vi "Open From Disk.vi"(8 "error in (no error)":errorcluster, 9 "Mode":T1, 10 "Path":path, 11 "Database Manager in":refnum<class "Database Manager.lvclass">) -> (0 "error out":errorcluster, 3 "Database Manager out":refnum<class "Database Manager.lvclass">)   [LabVIEW 2019, in "HierDAL Library.lvlib" / "Database.lvlib" / "Database Manager.lvclass"]
doc: "Opens a database on disk and initialises it.\n \n<b>Path</b> - Paths to the database on disk.\n<b>Mode</b> - The mode of operation (e.g., Create, Replace, Open, ReadOnly).\n <b>Create</b> - Creates a new database. If the database file already exists, it will be overwritten.\n <b>Replace</b> - Replaces the existing database with a new one.\n <b>Open</b> - Opens an existing database without modifying it.\n <b>Read Only</b> - Opens the database in read-only mode."
uses:
  Database Manager.lvclass
  Controls/Mode.ctl
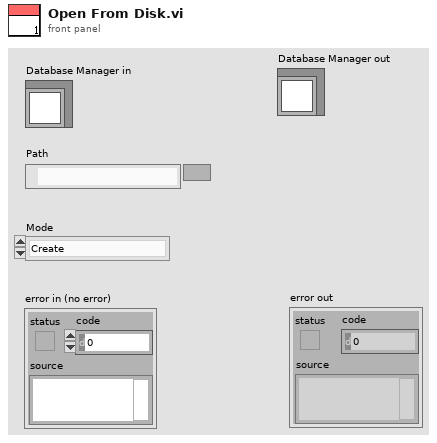
[diagram p1: front panel]
types:
  T1 = typedef "HierDAL Library.lvlib/Database.lvlib/Database Manager.lvclass/Mode.ctl" = enum16{"Create", "Replace", "Open", "Read Only"}
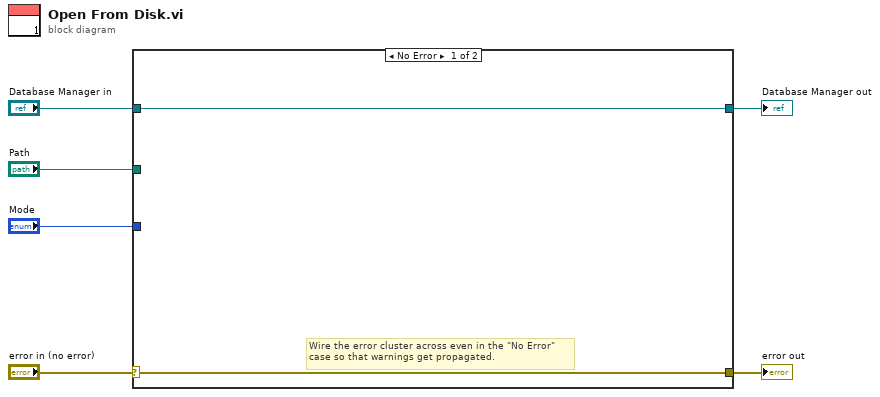
[diagram p0: block diagram]
diagram:
  n1 = case shown="No Error" "error in (no error)" {
    selector: "error in (no error)" -> [w7 w10]
    tunnel: [w7 w10] -> w5
    tunnel: [w8 w9] -> w3
    tunnel: "Database Manager in" -> [w8 w9]
    tunnel: "Path" -> [_ _]
    tunnel: "Mode" -> [_ _]
    frame No Error {
      # "Wire the error cluster across even in the \"No Error\"\ncase so that warnings get propagated."
    }
    frame Error {
    }
  }
  "error out" <- w5
  "Database Manager out" <- w3
